vi "Read pGames.vi"(8 "error in (no error)":errorcluster, 11 "bbPlayers in":refnum<class "bbPlayers.lvclass">) -> (0 "error out":errorcluster, 2 "pGames":i32, 3 "bbPlayers out":refnum<class "bbPlayers.lvclass">)   [LabVIEW 2020, in "ORM_Examples.lvlib" / "bbPlayers.lvclass"]
doc: "Read the current value for pGames."
uses:
  bbPlayers.lvclass
  bbPlayers.lvclass/bbPlayers.ctl
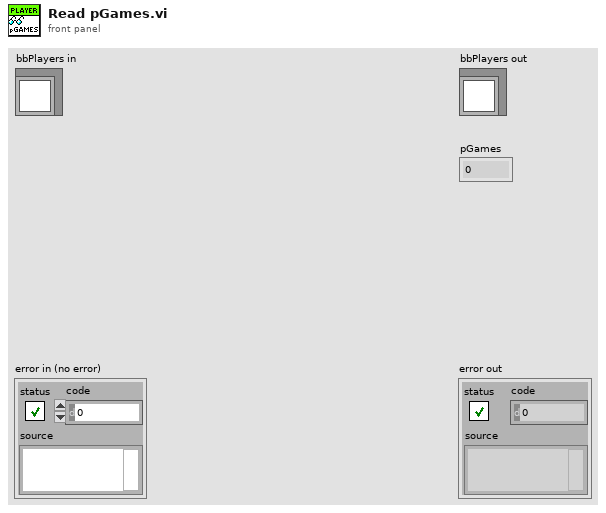
[diagram p1: front panel]
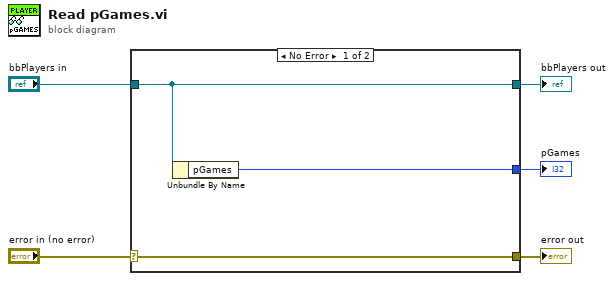
[diagram p0: block diagram]
diagram:
  n1 = case shown="No Error" "error in (no error)" {
    selector: "error in (no error)" -> [w8 w9]
    tunnel: [w8 w9] -> w4
    tunnel: [w7 w10] -> w2
    tunnel: "bbPlayers in" -> [w7 w10]
    tunnel: [w6 _] -> w1
    frame No Error {
      n2 = Unbundle By Name(w7) -> ("pGames"=w6:i32)
    }
    frame Error {
    }
  }
  "error out" <- w4
  "bbPlayers out" <- w2
  "pGames" <- w1
